vi "Get TreeItemArray.vi"(8 "error in (no error)":errorcluster, 11 "ClusterTree in":refnum<class "TreeLUT.lvclass">) -> (0 "error out":errorcluster, 2 "TreeItem Array":T1(array[cluster]), 3 "ClusterTree out":refnum<class "TreeLUT.lvclass">)   [LabVIEW 2017, in "TreeLUT.lvclass"]
uses:
  TreeLUT.lvclass
  HierElement.ctl
  <vilib>/Utility/Data Type/Type Definitions/Data Type.ctl
  TreeLUT.lvclass/TreeLUT.ctl
  <vilib>/Utility/Data Type/NI_Data Type.lvlib
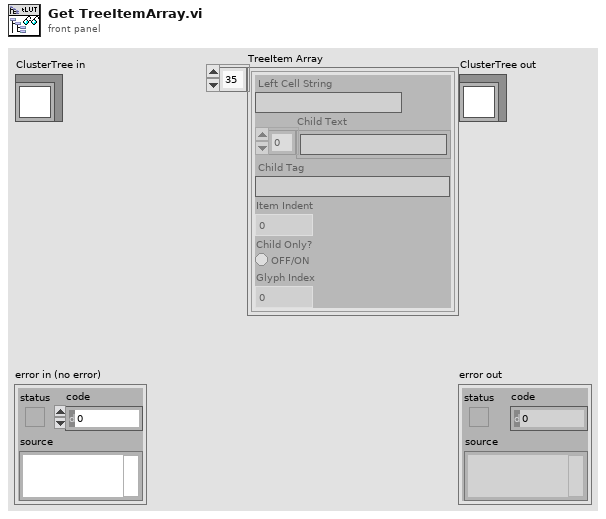
[diagram p1: front panel]
types:
  T1 = cluster{"Left Cell String":string, "Child Text":string[], "Child Tag":string, "Item Indent":i32, "Child Only?":bool, "Glyph Index":i32}[]
  T2 = typedef "TreeLUT.lvclass/HierElement.ctl" = cluster{"Parent":string, "Child":string, "ID":string, "Data Type":T3, "Indent":i32}
  T3 = typedef "NI_Data Type.lvlib/Data Type.ctl" = enum8{"Invalid Type", "Void", "I8", "I16", "I32", "I64", "U8", "U16", "U32", "U64", "Single Float", "Double Float", "Extended Float", "Single Complex", "Double Complex", "Extended Complex", "Enum U8", "Enum U16", "Enum U32", "Enum U64", "Single Float With Unit", "Double Float With Unit", "Extended Float With Unit", "Single Complex with Unit", "Double Complex with Unit", "Extended Complex with Unit", "Boolean", "String", "Path", "Picture", "Tag", "Array", "Cluster", "Variant", "LV Variant", "Waveform", "Timestamp", "Digital Waveform", "Digital Data", "ExpressData", "Refnum", "External Data", "VI", "Poly VI", "LabVIEW Class Instance", "Fixed Point"}
  T4 = cluster{"Left Cell String":string, "Child Text":string[], "Child Tag":string, "Item Indent":i32, "Child Only?":bool, "Glyph Index":i32}
  T5 = typedef "TreeLUT.lvclass/ClusterTree.ctl" = cluster{"LUT":variant, "Fields[]":string[], "Col[]":string[], "Type[]":T3[], "Indent[]":i32[]}
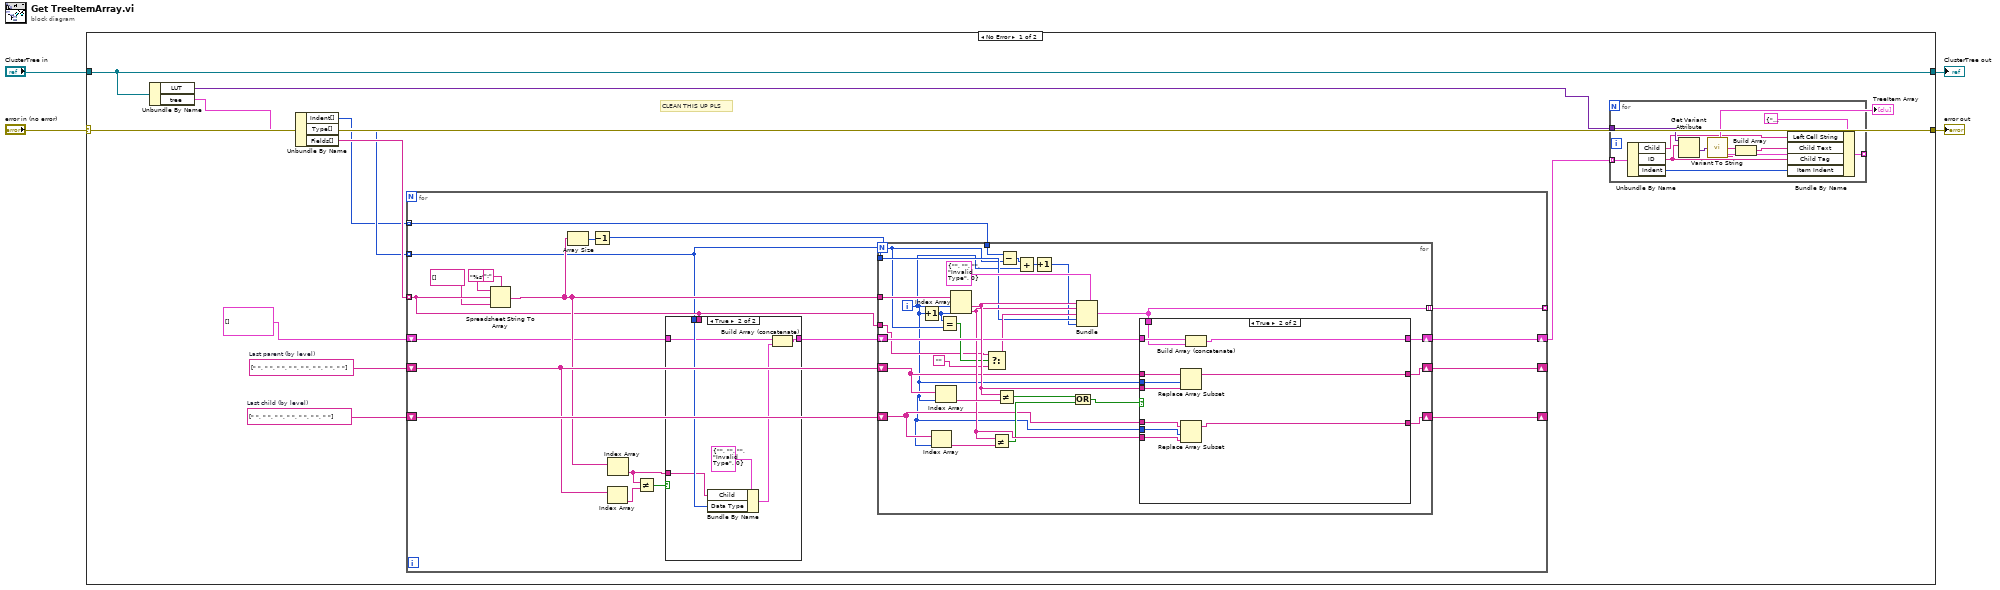
[diagram p0: block diagram]
diagram:
  n1 = case shown="No Error" "error in (no error)" {
    selector: "error in (no error)" -> [w16 w98]
    tunnel: [w16 w98] -> w3
    tunnel: [w15 w97] -> w1
    tunnel: "ClusterTree in" -> [w15 w97]
    frame No Error {
      w6 = string[] [" ", " ", " ", " ", " ", " ", " "]  # Last child (by level)
      w5 = string[] [" ", " ", " ", " ", " ", " ", " ", " "]  # Last parent (by level)
      # "CLEAN THIS UP PLS"
      n2 = Unbundle By Name(w15) -> ("LUT"=w12:variant, "tree"=w14:T5)
      n3 = Unbundle By Name(w14) -> ("Indent[]"=w8:i32[], "Type[]"=w9:T3[], "Fields[]"=w10:string[])
      n4 = for {
        tunnel: w10 -> [w35] mode=indexing
        tunnel: [w45] -> _ mode=indexing
        shift-right: [w43] -> w13
        shift-left: T2[] [] -> [w33]
        shift-right: [w44] -> _
        shift-left: w5 -> [w40]
        shift-right: [w41] -> _
        shift-left: w6 -> [w42]
        tunnel: w9 -> [w34] mode=indexing
        tunnel: w8 -> [w31] mode=indexing
        n5 = Spreadsheet String To Array(delimiter (Tab)=":" ("Delimiter"), format string="%s", spreadsheet string=w35, array type (2D Dbl)=string[] []) -> (array=w39:string[])
        n6 = Array Size(array=w39) -> (size(s)=w47:i32)
        n7 = Decrement(x=w47) -> (x-1=w46:i32)
        n8 = Index Array(array=w40) -> (element=w38:string)  [unwired: 1 in]
        n9 = Index Array(array=w39) -> (element=w36:string)  [unwired: 1 in]
        n10 = Not Equal?(x=w36, y=w38) -> (x != y?=w37:bool)
        n11 = case shown="True" w37 {
          tunnel: w36 -> [_ w52]
          tunnel: w35 -> [_ _]
          tunnel: w34 -> [_ w53]
          tunnel: w33 -> [w48 w51]
          tunnel: [w48 w49] -> w32
          frame False {
          }
          frame True {
            n12 = Bundle By Name(cluster=T2 {"Parent"="", "Child"="", "ID"="", "Data Type"=enum."Invalid Type", "Indent"=0} ("HierElement"), "Child"=w52, "Data Type"=w53) -> (w50:T2)
            n13 = Build Array (concatenate)(w51, w50) -> (w49:T2[])
          }
        }
        n14 = for {
          N: w46 -> [w59]
          tunnel: w39 -> [w82]
          tunnel: [w75] -> w45 mode=indexing
          shift-right: [w76] -> w43
          shift-left: w32 -> [w77]
          shift-right: [w78] -> w44
          shift-left: w40 -> [w68]
          shift-right: [w69] -> w41
          shift-left: w42 -> [w70]
          tunnel: w35 -> [w62]
          tunnel: w34 -> [w61]
          tunnel: w31 -> [w60]
          i -> [w57]
          n15 = Increment(x=w57) -> (x+1=w66:i32)
          n16 = Index Array(array=w70, index=w57) -> (element=w74:string)
          n17 = Index Array(array=w68, index=w57) -> (element=w80:string)
          n18 = Equal?(x=w66, y=w59) -> (x = y?=w65:bool)
          n19 = Index Array(array=w82, index #1=w57, index #2=w66) -> (element #1=w79:string, element #2=w73:string)
          n20 = Select(t=w62, s=w65, f="") -> (s? t:f=w64:string)
          n21 = Not Equal?(x=w73, y=w74) -> (x != y?=w71:bool)
          n22 = Not Equal?(x=w79, y=w80) -> (x != y?=w72:bool)
          n23 = Subtract(x=w60, y=w59) -> (x-y=w58:i32)
          n24 = Add(x=w58, y=w57) -> (x+y=w56:i32)
          n25 = Increment(x=w56) -> (x+1=w55:i32)
          n26 = Compound Arithmetic op=OR(w72, w71) -> (w67:bool)
          n27 = Bundle(cluster=T2 {"Parent"="", "Child"="", "ID"="", "Data Type"=enum."Invalid Type", "Indent"=0} ("HierElement"), "Parent"=w79, "Child"=w73, "ID"=w64, "Data Type"=w61, "Indent"=w55) -> (w75:T2)
          n28 = case shown="True" w67 {
            tunnel: w68 -> [w85 w96]
            tunnel: w79 -> [_ w95]
            tunnel: w57 -> [_ w94]
            tunnel: [w85 w93] -> w78
            tunnel: w77 -> [w84 w92]
            tunnel: [w84 w91] -> w76
            tunnel: w75 -> [_ w90]
            tunnel: w57 -> [_ w89]
            tunnel: w73 -> [_ w88]
            tunnel: w70 -> [w83 w87]
            tunnel: [w83 w86] -> w69
            frame False {
            }
            frame True {
              n29 = Replace Array Subset(array=w96, new element=w95, index=w94) -> (w93:string[])
              n30 = Replace Array Subset(array=w87, new element=w88, index=w89) -> (w86:string[])
              n31 = Build Array (concatenate)(w92, w90) -> (w91:T2[])
            }
          }
        }
      }
      n32 = for {
        tunnel: w13 -> [w27] mode=indexing
        tunnel: w12 -> [w26]
        tunnel: [w24] -> w11 mode=indexing
        n33 = Unbundle By Name(w27) -> ("Child"=w23:string, "ID"=w22:string, "Indent"=w20:i32)
        n34 = Get Variant Attribute(Variant=w26, name=w22) -> (value=w19:variant)  [unwired: 2 in, 3 out]
        n35 = call "Variant To String.vi"("Variant"=w19) -> ("String"=w18:string, "Data Type"=w17:string)  [unwired: 13 in]
        n36 = Build Array(w18, w17) -> (w21:string[])
        n37 = Bundle By Name(cluster=T4 {"Left Cell String"="", "Child Text"=[], "Child Tag"="", "Item Indent"=0, "Child Only?"=FALSE, "Glyph Index"=0} ("element"), "Left Cell String"=w23, "Child Text"=w21, "Child Tag"=w22, "Item Indent"=w20) -> (w24:T4)
      }
      "TreeItem Array" <- w11
    }
    frame Error {
    }
  }
  "error out" <- w3
  "ClusterTree out" <- w1
